vi "test_Copy LogFile from Target.vi"(8 "error in (no error)":errorcluster, 11 "TestCase in":refnum<class "Telemetry System Tests.lvclass">) -> (0 "error out":errorcluster, 3 "TestCase out":refnum<class "Telemetry System Tests.lvclass">)   [LabVIEW 2019, in "Telemetry System Tests.lvclass"]
uses:
  Telemetry System Tests.lvclass
  b15e678b-00b4-460c-84a3-511904b6b81c.vi
  <vilib>/addons/_JKI Toolkits/VI Tester/TestCase.llb/TestCase.lvclass
  TLCD Test/TLCD Test.lvclass
  C:/Program Files (x86)/National Instruments/LabVIEW 2019/vi.lib/addons/_JKI Toolkits/VI Tester/TestCase.llb/TestCase.lvclass
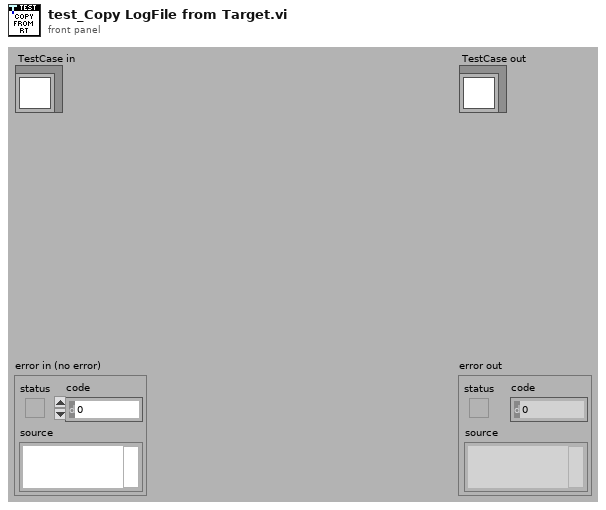
[diagram p1: front panel]
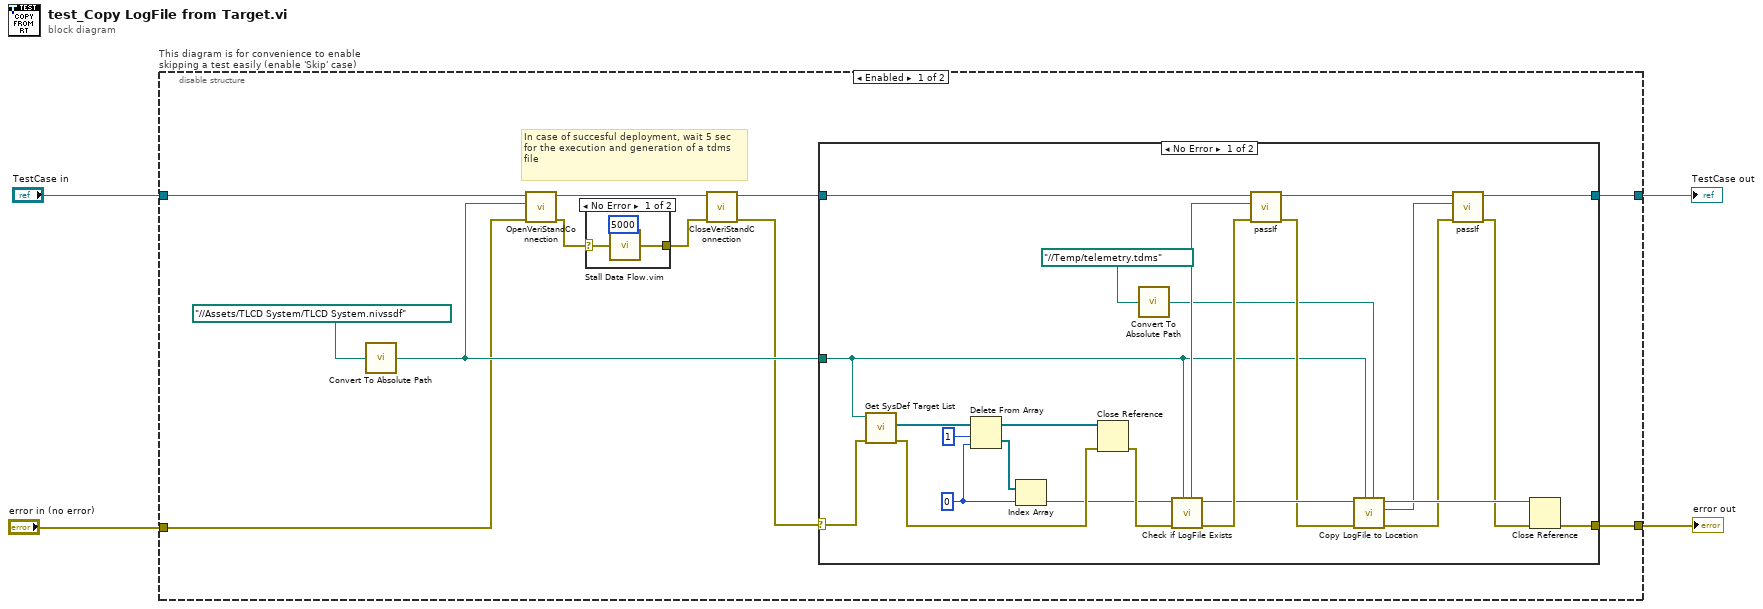
[diagram p0: block diagram]
diagram:
  n1 = disable-structure "This diagram is for convenience to enable skipping a test easily (enable 'Skip' case)" shown="Enabled" {
    disable-tunnel: "TestCase in" -> [w12 w49]
    disable-tunnel: [w13 w47] -> w1
    disable-tunnel: [w14 w48] -> w3
    disable-tunnel: "error in (no error)" -> [w10 w46]
    frame Enabled {
      # "In case of succesful deployment, wait 5 sec for the execution and generation of a tdms file"
      n2 = call "Convert To Absolute Path.vi"("System Definition File Path"=path "../../Assets/TLCD System/TLCD System.nivssdf" ("relative base path")) -> ("Absolute path"=w11:path)
      n3 = call-dynamic "OpenVeriStandConnection.vi"("error in (no error)"=w10, "System Definition File"=w11, "VeriStand Test Case in"=w12) -> ("error out"=w6:errorcluster, "VeriStand Test Case out"=w7:refnum<class "Telemetry System Tests.lvclass">)  [unwired: 6 in, 1 out]
      n4 = case shown="No Error" w6 {
        selector: w6 -> [w18 w19]
        tunnel: [w16 w19] -> w5
        frame No Error {
          n5 = call "Stall Data Flow.vim"("value in"=w18, "milliseconds to wait"=u32 5000) -> ("value out"=w16:errorcluster)  [unwired: 1 out]
        }
        frame Error {
        }
      }
      n6 = call-dynamic "CloseVeriStandConnection.vi"("error in (no error)"=w5, "VeriStand Test Case in"=w7) -> ("error out"=w8:errorcluster, "VeriStand Test Case out"=w9:refnum<class "Telemetry System Tests.lvclass">)  [unwired: 8 in]
      n7 = case shown="No Error" w8 {
        selector: w8 -> [w25 w45]
        tunnel: [w43 w45] -> w14
        tunnel: [w20 w44] -> w13
        tunnel: w11 -> [w27 _]
        tunnel: w9 -> [w26 w44]
        frame No Error {
          w39 = 0 ("index")
          n8 = call "Get SysDef Target List.vi"("error in (no error)"=w25, "System Definition Path"=w27) -> ("error out"=w37:errorcluster, "Target List"=w42:refnum<k24>[])  [unwired: 8 in]
          n9 = Delete From Array(array=w42, length=1, index=w39) -> (deleted portion=w40:refnum<k24>[], array with subset deleted=w38:refnum<k24>[])
          n10 = Index Array(array=w40, index=w39) -> (element=w35:refnum<k24>)
          n11 = Close Reference(reference=w38, error in (no error)=w37) -> (error out=w36:errorcluster)
          n12 = call "Convert To Absolute Path.vi"("System Definition File Path"=path "../../Temp/telemetry.tdms" ("relative base path")) -> ("Absolute path"=w28:path)
          n13 = call "Check if LogFile Exists.vi"("System Definition Path"=w27, "error in (no error)"=w36, "Target Refnum in"=w35) -> ("error out"=w34:errorcluster, "Target Refnum out"=w32:refnum<k24>, "LogFile Exists?"=w33:bool)  [unwired: 6 in]
          n14 = call-dynamic "passIf.vi"("error in (no error)"=w34, "pass"=w33, "TestCase in"=w26) -> ("error out"=w31:errorcluster, "TestCase out"=w24:refnum<class "Telemetry System Tests.lvclass">)  [unwired: 7 in]
          n15 = call "Copy LogFile to Location.vi"("Local Save path"=w28, "System Definition Path"=w27, "error in (no error)"=w31, "Target Refnum in"=w32) -> ("error out"=w22:errorcluster, "File Succesfuly copied"=w23:bool, "Target Refnum out"=w30:refnum<k24>)  [unwired: 5 in]
          n16 = call-dynamic "passIf.vi"("error in (no error)"=w22, "pass"=w23, "TestCase in"=w24) -> ("error out"=w21:errorcluster, "TestCase out"=w20:refnum<class "Telemetry System Tests.lvclass">)  [unwired: 7 in]
          n17 = Close Reference(reference=w30, error in (no error)=w21) -> (error out=w43:errorcluster)
        }
        frame Error {
        }
      }
    }
    frame Disabled {
      # "skip test result while test is under development"
      n18 = call <vilib>:"skip.vi"("error in (no error)"=w46, "TestCase in"=w49) -> ("error out"=w48:errorcluster, "TestCase out"=w47:refnum<class "Telemetry System Tests.lvclass">)  [unwired: 8 in]
    }
  }
  "error out" <- w3
  "TestCase out" <- w1
